vi "SetServoToPosition.vi"(3 "error in (no error)":errorcluster, 4 "RF LF":dbl caption="Angle", 5 "VISA resource name":refnum<visa-resource-name>) -> (0 "error out":errorcluster, 1 "RF LF 2":dbl caption="Angle", 2 "VISA resource name out":refnum<visa-resource-name>)   [LabVIEW 2014]
uses:
  <vilib>/Instr/_visa.llb/VISA Configure Serial Port (Instr).vi
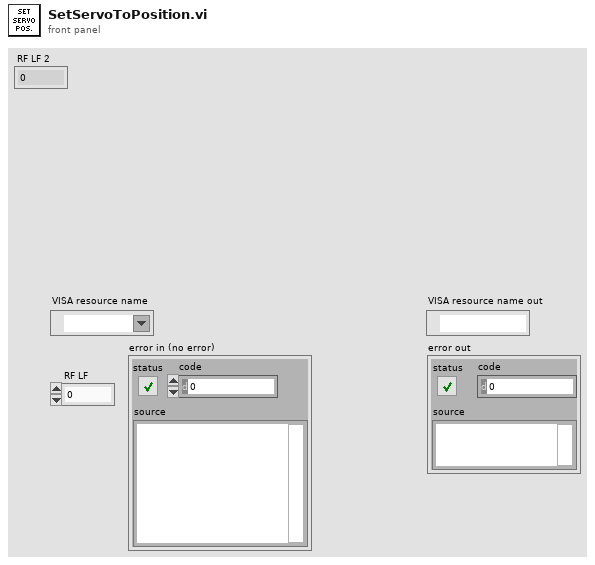
[diagram p1: front panel]
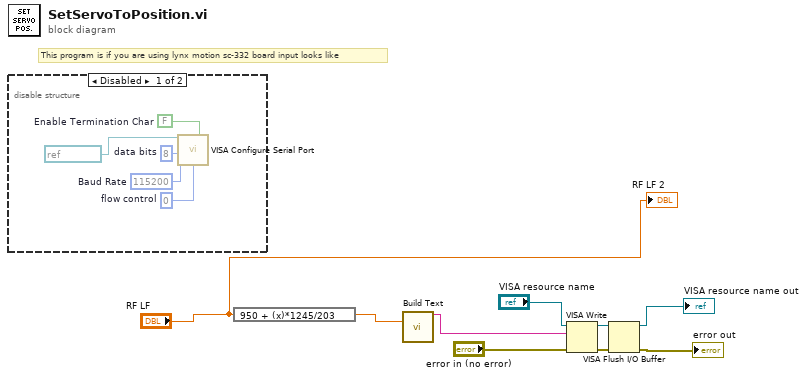
[diagram p0: block diagram]
diagram:
  # "This program is if you are using lynx motion sc-332 board input looks like"
  n1 = disable-structure shown="Disabled" {
    frame Disabled {
      w13 = u32 115200  # Baud Rate
      w12 = u16 0  # flow control
      w14 = u16 8  # data bits
      w11 = FALSE  # Enable Termination Char
      n2 = call-poly "VISA Configure Serial Port"("VISA resource name"=refnum<visa-resource-name> "COM3", "Enable Termination\nChar (T)"=w11, "baud rate (9600)"=w13, "data bits (8)"=w14, "flow control (0:none)"=w12) -> ()  [unwired: 9 in, 2 out]
    }
    frame Enabled {
    }
  }
  n3 = expression code="950 + (x)*1245/203"("RF LF") -> (w4:dbl)
  n4 = call "Build Text"("RF angle"=w4) -> ("Result"=w9:string)  [unwired: 13 in, 1 out]
  n5 = VISA Write(VISA resource name="VISA resource name", write buffer=w9, error in (no error)="error in (no error)") -> (VISA resource name out=w6:refnum<visa-resource-name>, error out=w7:errorcluster)  [unwired: 1 out]
  n6 = VISA Flush I/O Buffer(VISA resource name=w6, error in (no error)=w7) -> (VISA resource name out=→"VISA resource name out":refnum<visa-resource-name>, error out=→"error out":errorcluster)  [unwired: 1 in]
  "RF LF 2" <- "RF LF"
